vi "DataAnalysis.vi"() -> ()   [LabVIEW 2015]
uses:
  <vilib>/Utility/file.llb/Read Delimited Spreadsheet (DBL).vi
panel:
  out "Histogram":dynamicdata(graph)=[{"t0"=timestamp(23.05 s since 1904-01-01), "dt"=6.1, "Y"=[0.0, 0.0, 0.0, 1.0, 3.0, 16.0, 22.0, 7.0, 6.0, 5.0], "attributes"=variant("NI_ChannelName"=variant(string " (Histogram)"), "NI_ExpIsRelativeTime"=variant(bool TRUE), "NI_ExpStartTimeStamp"=variant(timestamp timestamp(3531262931.7832003 s since 1904-01-01)), "NI_ExpTimeStamp"=variant(timestamp timestamp(3531262931.7832003 s since 1904-01-01)), "NI_ExpXDimension"=variant(string "BIN"), "NI_OriginalChannelName"=variant(string ""))}]
  in  "file path (dialog if empty) 2":path=path "C:/Users/minor6th/Desktop/PHYS434/week8/WaterCalibration"
  in  "file path (dialog if empty)":path=path "C:/Users/minor6th/Desktop/PHYS434/week8/DecayRateData"
  out "Waveform Graph":dbl[][](graph)=[[0.0, 24.0, 20.0, 18.0, 18.0, 24.0, 21.0, 22.0, 27.0, 19.0, 22.0, 23.0, 11.0, 32.0, 19.0, 23.0, 21.0, 11.0, 20.0, 14.0, 20.0, 13.0, 14.0, 11.0, 10.0, 13.0, 8.0, 15.0, 8.0, 16.0, 24.0, 22.0, 14.0, 11.0, 13.0, 14.0, 18.0, 16.0, 12.0, 21.0, 18.0, 20.0, 16.0, 14.0, 10.0, 15.0, 17.0, 17.0, 18.0, 21.0, 16.0, 9.0, 13.0, 16.0, 16.0, 18.0, 16.0, 10.0, 14.0, 13.0, 13.0, 12.0, 8.0, 11.0, 16.0, 7.0, 13.0, 8.0, 13.0, 12.0, 10.0, 8.0, 13.0, 14.0, 9.0, 10.0, 17.0, 10.0, 7.0, 11.0, 16.0, 13.0, 13.0, 11.0, 10.0, 3.0, 17.0, 7.0, 6.0, 6.0, 12.0, 13.0, 5.0, 5.0, 13.0, 9.0, 8.0, 10.0, 13.0, 5.0, 10.0, 14.0, 8.0, 10.0, 9.0, 12.0, 6.0, 11.0, 6.0, 8.0, 5.0, 7.0, 10.0, 9.0, 11.0, 6.0, 9.0, 4.0, 6.0, 14.0, 11.0, 7.0, 5.0, 9.0, 9.0, 7.0, 8.0, 2.0, 4.0, 7.0, 8.0, 3.0, 8.0, 12.0, 8.0, 2.0, 8.0, 10.0, 9.0, 6.0, 6.0, 7.0, 11.0, 9.0, 5.0, 6.0, 9.0, 4.0, 3.0, 8.0, 6.0, 3.0, 4.0, 5.0, 8.0, 7.0, 3.0, 5.0, 5.0, 3.0, 6.0, 3.0, 5.0, 1.0, 7.0, 8.0, 1.0, 7.0, 5.0, 5.0, 5.0, 4.0, 5.0, 6.0, 2.0, 5.0, 4.0, 6.0, 4.0, 1.0, 2.0, 1.0, 2.0, 1.0, 6.0, 5.0, 4.0, 4.0, 3.0, 3.0, 4.0, 2.0, 2.0, 5.0, 3.0, 4.0, 5.0, 3.0, 3.0, 8.0, 7.0, 3.0, 2.0, 4.0, 4.0, 2.0, 1.0, 1.0, 2.0, 1.0, 8.0, 2.0, 0.0, 1.0, 4.0, 1.0, 3.0, 2.0, 5.0, 1.0, 3.0, 2.0, 7.0, 5.0, 1.0, 1.0, 3.0, 3.0, 1.0, 3.0, 2.0, 5.0, 4.0, 0.0, 1.0, 2.0, 3.0, 3.0, 2.0, 2.0, 1.0, 0.0, 5.0, 3.0, 3.0, 1.0, 2.0, 4.0, 2.0, 6.0, 4.0, 1.0, 2.0, 1.0, 2.0, 3.0, 3.0, 1.0, 3.0, 3.0, 4.0, 1.0, 3.0, 2.0, 1.0, 3.0, 7.0, 4.0, 1.0, 1.0, 2.0, 2.0, 6.0, 5.0, 3.0, 0.0, 1.0, 3.0, 1.0, 1.0, 2.0, 1.0, 2.0, 1.0, 0.0, 0.0, 1.0, 5.0, 1.0, 3.0, 2.0, 3.0, 1.0, 2.0, 3.0, 6.0, 2.0, 1.0, 2.0, 1.0, 3.0], [31.74020898013987, 28.176845478599716, 26.092562167519645, 24.613807087094756, 23.466834098668187, 22.529713939424255, 21.737407680491742, 21.051093775946356, 20.44573202218453, 19.90422543371824, 19.41437960917392, 18.967190774346818, 18.555821446949267, 18.17495680294087, 17.820383641788794, 17.488705515497713, 17.17714437383256, 16.883398993028095, 16.605541733355494, 16.341941809914715, 16.091207304045383, 15.85214067735069, 15.623704182748043, 15.404992642630532, 15.195211787766311, 14.993660847263527, 14.79971842606028, 14.612830952137301, 14.43250315192563, 14.258290141129692, 14.089790812882711, 13.926642276099301, 13.768515149815357, 13.6151095602836, 13.466151718494075, 13.321390979886928, 13.180597307087737, 13.043559071025811, 12.910081137772067, 12.77998319760809, 12.653098300484999, 12.529271567967953, 12.40835905676795, 12.290226752957096, 12.174749679208617, 12.061811100174964, 11.951301813365717, 11.84311951460404, 11.73716822903225, 11.633357799481018, 11.531603425646608, 11.431825247855159, 11.333947970626468, 11.237900521344272, 11.143615740256791, 11.051030098438787, 10.960083440688322, 10.870718750775268, 10.782881936815102, 10.696521634614328, 10.611589027328591, 10.528037679716363, 10.445823385744006, 10.36490402808704, 10.28523944864719, 10.206791328826512, 10.129523078896455, 10.053399735537823, 9.978387866845878, 9.904455484189384, 9.831571960290603, 9.75970795309695, 9.688835334811301, 9.618927125862683, 9.54995743319887, 9.481901392733562, 9.414735115562507, 9.348435637584771, 9.28298087240546, 9.218349567148834, 9.154521261065383, 9.091476246605453, 9.029195532952144, 8.967660811649694, 8.906854424290941, 8.846759332125657, 8.787359087400546, 8.728637806329061, 8.670580143603729, 8.61317126834183, 8.556396841311653, 8.500242993468419, 8.444696305625257, 8.389743789179192, 8.335372867884871, 8.28157136063237, 8.228327464981703, 8.175629741715966, 8.123467100012931, 8.071828783504316, 8.020704356909846, 7.970083693413471, 7.919956962614378, 7.870314619067358, 7.82114739138342, 7.772446271847002, 7.724202506484289, 7.676407585633569, 7.629053234952153, 7.58213140679436, 7.535634272040625, 7.489554212203075, 7.443883811996784, 7.398615852129296, 7.353743302490329, 7.309259315567033, 7.265157220201218, 7.221430515564862, 7.178072865412105, 7.135078092600452, 7.092440173779323, 7.050153234296886, 7.0082115434342995, 6.966609509654518, 6.925341676171229, 6.884402716648765, 6.843787431083911, 6.803490741825954, 6.763507689771359, 6.72383343072579, 6.68446323183889, 6.6453924682646175, 6.6066166198434075, 6.5681312680389965, 6.529932092853414, 6.492014869931154, 6.454375467801583, 6.417009845092252, 6.379914048011415, 6.343084207786887, 6.306516538264987, 6.270207333553117, 6.23415296580788, 6.198349883008632, 6.1627946068838355, 6.127483730917447, 6.092413918318925, 6.057581900175137, 6.022984473624092, 5.98861850007961, 5.954480903521471, 5.920568668836495, 5.88687884023966, 5.853408519702498, 5.820154865490622, 5.7871150906794355, 5.7542864617935265, 5.721666297387856, 5.689251966810843, 5.657040888887423, 5.625030530674849, 5.593218406291271, 5.561602075758856, 5.530179143868736, 5.4989472590823425, 5.46790411251277, 5.4370474368552095, 5.406375005433802, 5.375884631212102, 5.345574165854487, 5.315441498853033, 5.28548455658165, 5.255701301517547, 5.226089731346292, 5.196647878197837, 5.167373807824333, 5.138265618865262, 5.1093214420980075, 5.0805394397175405, 5.051917804637924, 5.023454759793822, 4.995148557522043, 4.966997478870326, 4.9389998329861555, 4.911153956527414, 4.883458213043923, 4.8559109924171935, 4.828510710285627, 4.801255807513371, 4.774144749630068, 4.74717602635792, 4.720348151051439, 4.6936596602608915, 4.667109113208426, 4.6406950913515175, 4.614416197917308, 4.588271057436941, 4.562258315367217, 4.53637663761765, 4.5106247101794, 4.485001238666882, 4.459504948012182, 4.4341345820139395, 4.40888890298811, 4.383766691411438, 4.358766745586763, 4.333887881242845, 4.309128931250598, 4.284488745273848, 4.259966189441911, 4.235560146044008, 4.211269513238221, 4.1870932047240785, 4.163030149480619, 4.139079291446251, 4.11523958928592, 4.091510016078246, 4.067889559068135, 4.044377219404851, 4.02097201190918, 3.997672964782396, 3.974479119402531, 3.9513895300624426, 3.9284032637660857, 3.905519399966579, 3.8827370303843054, 3.8600552587449783, 3.83747320061957, 3.814989983184205, 3.7926047450164333, 3.770316635906056, 3.7481248166659498, 3.726028458950168, 3.7040267450356623, 3.6821188676694874, 3.660304029879626, 3.6385814448149176, 3.6169503355486086, 3.5954099349401076, 3.573959485445812, 3.552598238988139, 3.5313254567663535, 3.510140409132873, 3.4890423754186486, 3.4680306438094703, 3.4471045111786225, 3.426263282970467, 3.4055062730403733, 3.384832803516474, 3.3642422046978027, 3.3437338149014977, 3.323306980317284, 3.3029610549347126, 3.2826954003685387, 3.2625093857568572, 3.242402387651964, 3.2223737898966647, 3.2024229835296865, 3.182549366618332, 3.162752344229375, 3.1430313282617135, 3.123385737359058, 3.103814996815345, 3.0843185384728713, 3.064895800605882, 3.045546227847808, 3.0262692710675765, 3.007064387318678, 2.987931039708201, 2.9688686973022413, 2.949876835089526, 2.930954933835892, 2.9121024800333544, 2.893318965798244, 2.8746038888129988, 2.8559567522170255, 2.837377064541215, 2.8188643396424595, 2.8004180965945125, 2.7820378596516093, 2.76372315815388, 2.745473526447313, 2.727288503832824, 2.709167634478945, 2.6911104673636146, 2.673116556215973, 2.655185459414497, 2.637316739972448, 2.6195099654214573, 2.60176470780425, 2.5840805435582297, 2.566457053486374, 2.5488938226990285, 2.531390440541145, 2.5139465005413513, 2.4965616003610194, 2.4792353417215054, 2.461967330375046, 2.444757176017447, 2.427604492273531, 2.4105088966171024]]
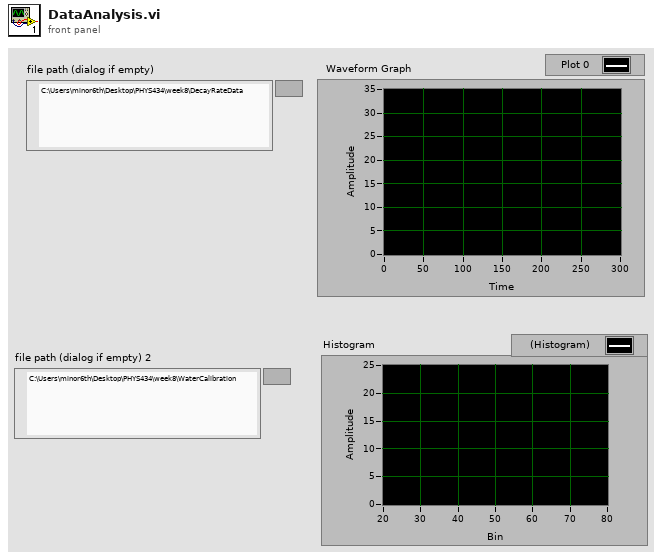
[diagram p1: front panel]
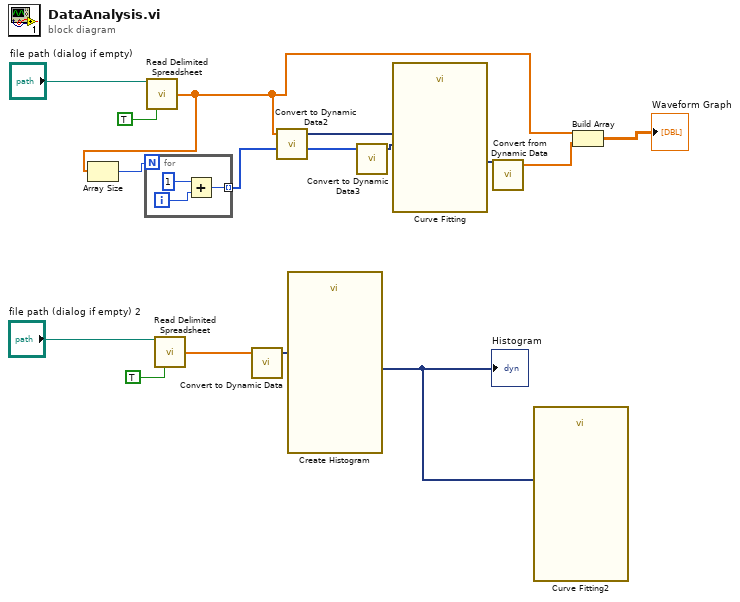
[diagram p0: block diagram]
diagram:
  n1 = call-poly <vilib>:"Read Delimited Spreadsheet.vi"("file path (dialog if empty)"="file path (dialog if empty)", "transpose? (F)"=TRUE) -> ("first row"=w2:dbl[])  [unwired: 8 in, 5 out]
  n2 = Array Size(array=w2) -> (size(s)=w9:i32)
  n3 = for {
    N: w9 -> [_]
    tunnel: [w16] -> w8 mode=indexing
    i -> [w18]
    n4 = Add(x=1, y=w18) -> (x+y=w16:i32)
  }
  n5 = call-poly <vilib>:"Read Delimited Spreadsheet.vi"("file path (dialog if empty)"="file path (dialog if empty) 2", "transpose? (F)"=TRUE) -> ("first row"=w10:dbl[])  [unwired: 8 in, 5 out]
  n6 = call "Convert to Dynamic Data"("Array"=w10) -> ("Dynamic Data Type"=w11:dynamicdata)  [unwired: 3 in]
  n7 = call "Convert to Dynamic Data2"("Array"=w2) -> ("Dynamic Data Type"=w6:dynamicdata)  [unwired: 3 in]
  n8 = call "Create Histogram"("Signal"=w11) -> ("Histogram"=w1:dynamicdata)  [unwired: 9 in, 1 out]
  "Histogram" <- w1
  n9 = call "Convert to Dynamic Data3"("Array"=w8) -> ("Dynamic Data Type"=w7:dynamicdata)  [unwired: 3 in]
  n10 = call "Curve Fitting"("Locations"=w7, "Signals"=w6) -> ("best fit"=w5:dynamicdata)  [unwired: 6 in, 3 out]
  n11 = call "Convert from Dynamic Data"("Dynamic Data Type"=w5) -> ("Array"=w3:dbl[])  [unwired: 3 in]
  n12 = call "Curve Fitting2"("Signals"=w1) -> ()  [unwired: 6 in, 5 out]
  n13 = Build Array(w2, w3) -> (→"Waveform Graph":dbl[][])
